vi "cRIO MC Test.vi"() -> ()   [LabVIEW 2009]
uses:
  Remote Control/Motor Command.ctl
  <vilib>/Platform/TimedLoop/XDataNode/wakeup.ctl
  <vilib>/Platform/TimedLoop/XDataNode/XDNodeRunTimeDep.lvlib
  <vilib>/Platform/TimedLoop/XDataNode/nitl_modes.ctl
  <vilib>/Platform/TimedLoop/XDataNode/timing_clust.ctl
  <vilib>/Platform/TimedLoop/XDataNode/XDataNode.xnode
  <vilib>/Platform/TimedLoop/XDataNode/loadlvalarms.vi
  TypeDefs/State Machine/Main State.ctl
  TypeDefs/Queue TypeDefs/Motor State.ctl
  TypeDefs/Queue TypeDefs/Motor Instruction.ctl
  Remote Control/Message Type.ctl
  Remote Control/Control Message.ctl
panel:
  in  "STOP":bool
  out "VI":bool
  in  "MC CMD \n INPUT":T1
  out "UDP HB":bool
  out "Main HB":bool
  out "Motor State":T2=enum."Initialize"
  out "MC HB":bool
  in  "GO":bool
  out "Saftey OFF":bool
  in  "Control Message":T3
  out "Motor Queue":refnum<queue>
  out "RC/!Run":bool
  out "Main State":T4
  in  "RC Command Buffer":T1
  in  "Motors Init Complete":bool
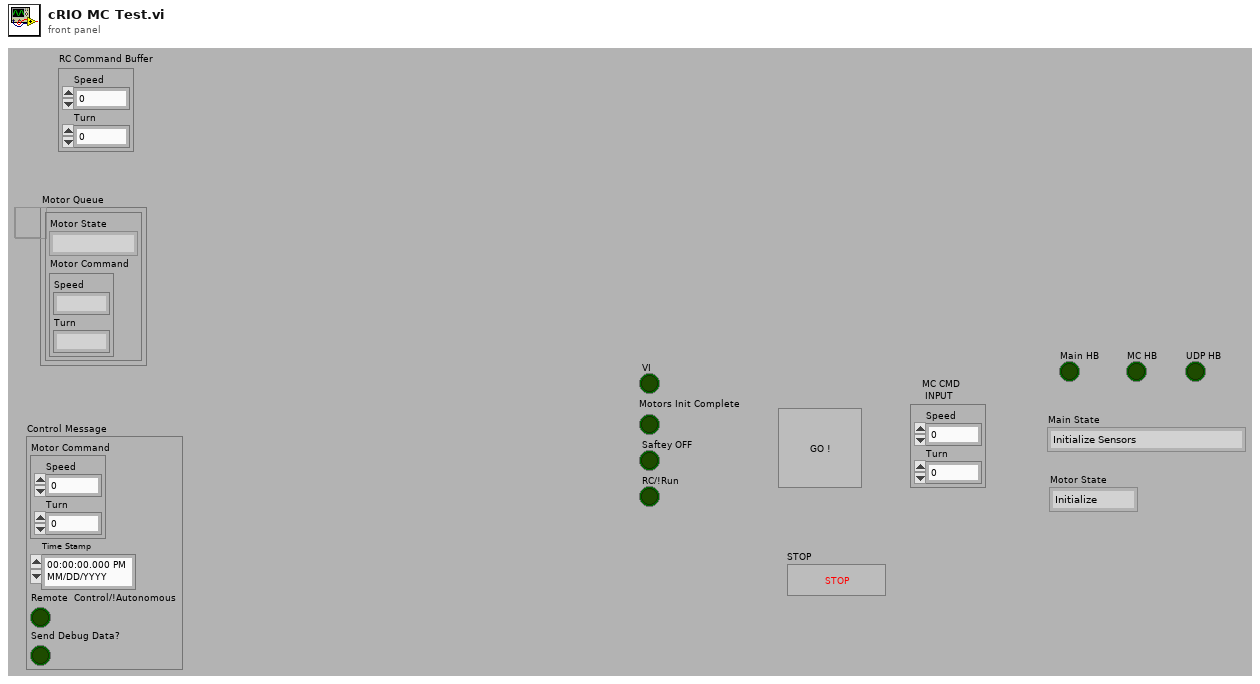
[diagram p1: front panel]
types:
  T1 = typedef "Motor Command.ctl" = cluster{"Speed":i16, "Turn":i16}
  T2 = typedef "Motor State.ctl" = enum16{"Wait", "Initialize", "Check FET", "Run", "Stop"}
  T3 = typedef "Control Message.ctl" = cluster{"Motor Command":T1, "Time Stamp":timestamp, "Remote  Control/!Autonomous":bool, "Send Debug Data?":bool}
  T4 = typedef "Main State.ctl" = enum16{"Initialize Sensors", "Initialize Motors", "Wait for GO", "Run", "Remote Control", "Stop"}
  T5 = typedef "Motor Instruction.ctl" = cluster{"Motor State":T2, "Motor Command":T1}
  T6 = typedef "UDP Base.ctl" = cluster{"UDP Session":refnum<k16>, "UDP Socket Params":T7}
  T7 = typedef "UDP Socket Params.ctl" = cluster{"Local Port":u16, "Read Timeout":i32, "Write Timeout":i32}
  T8 = typedef "XDNodeRunTimeDep.lvlib/timing_clust.ctl" = cluster{"Expected End [f-1]":u64, "Actual End [f-1]":u64, "Finished Late? [f-1]":bool, "Expected End [i-1]":u64, "Actual End [i-1]":u64, "Finished Late? [i-1]":bool, "Expected Start [i]":u64, "Actual Start [i]":u64, "Expected Start [f]":u64, "Actual Start [f]":u64, "Source Name":string, "Structure Name":string, "Period":i64, "Deadline":i64, "Offset":i64, "Start":i64, "Priority":i32, "Timeout":i32, "Mode":T9, "Wakeup Reason":T10, "Error":errorcluster, "Source Type":string, "Secondary Source Type":string, "Global End Time":u64, "Global Start Time":u64, "Frame Duration":u64, "Iteration Duration":u64, "Assigned CPU":i32, "I/O Scan Engine Mode":u32}
  T9 = typedef "XDNodeRunTimeDep.lvlib/nitl_modes.ctl" = enum32{"No Change", "Process missed periods, maintain original phase", "Discard missed periods, maintain original phase", "Process missed periods, ignore original phase", "Discard missed periods, ignore original phase"}
  T10 = typedef "XDNodeRunTimeDep.lvlib/wakeup.ctl" = enum32{"Normal", "Aborted", "Asynchronous wakeup", "Timing source error", "Timed loop error", "Timeout"}
  T11 = typedef "Message Type.ctl" = enum16{"Motor Command", "Debug Data"}
  T12 = typedef "UDP Network Location.ctl" = cluster{"IP Address":string, "Port":u16}
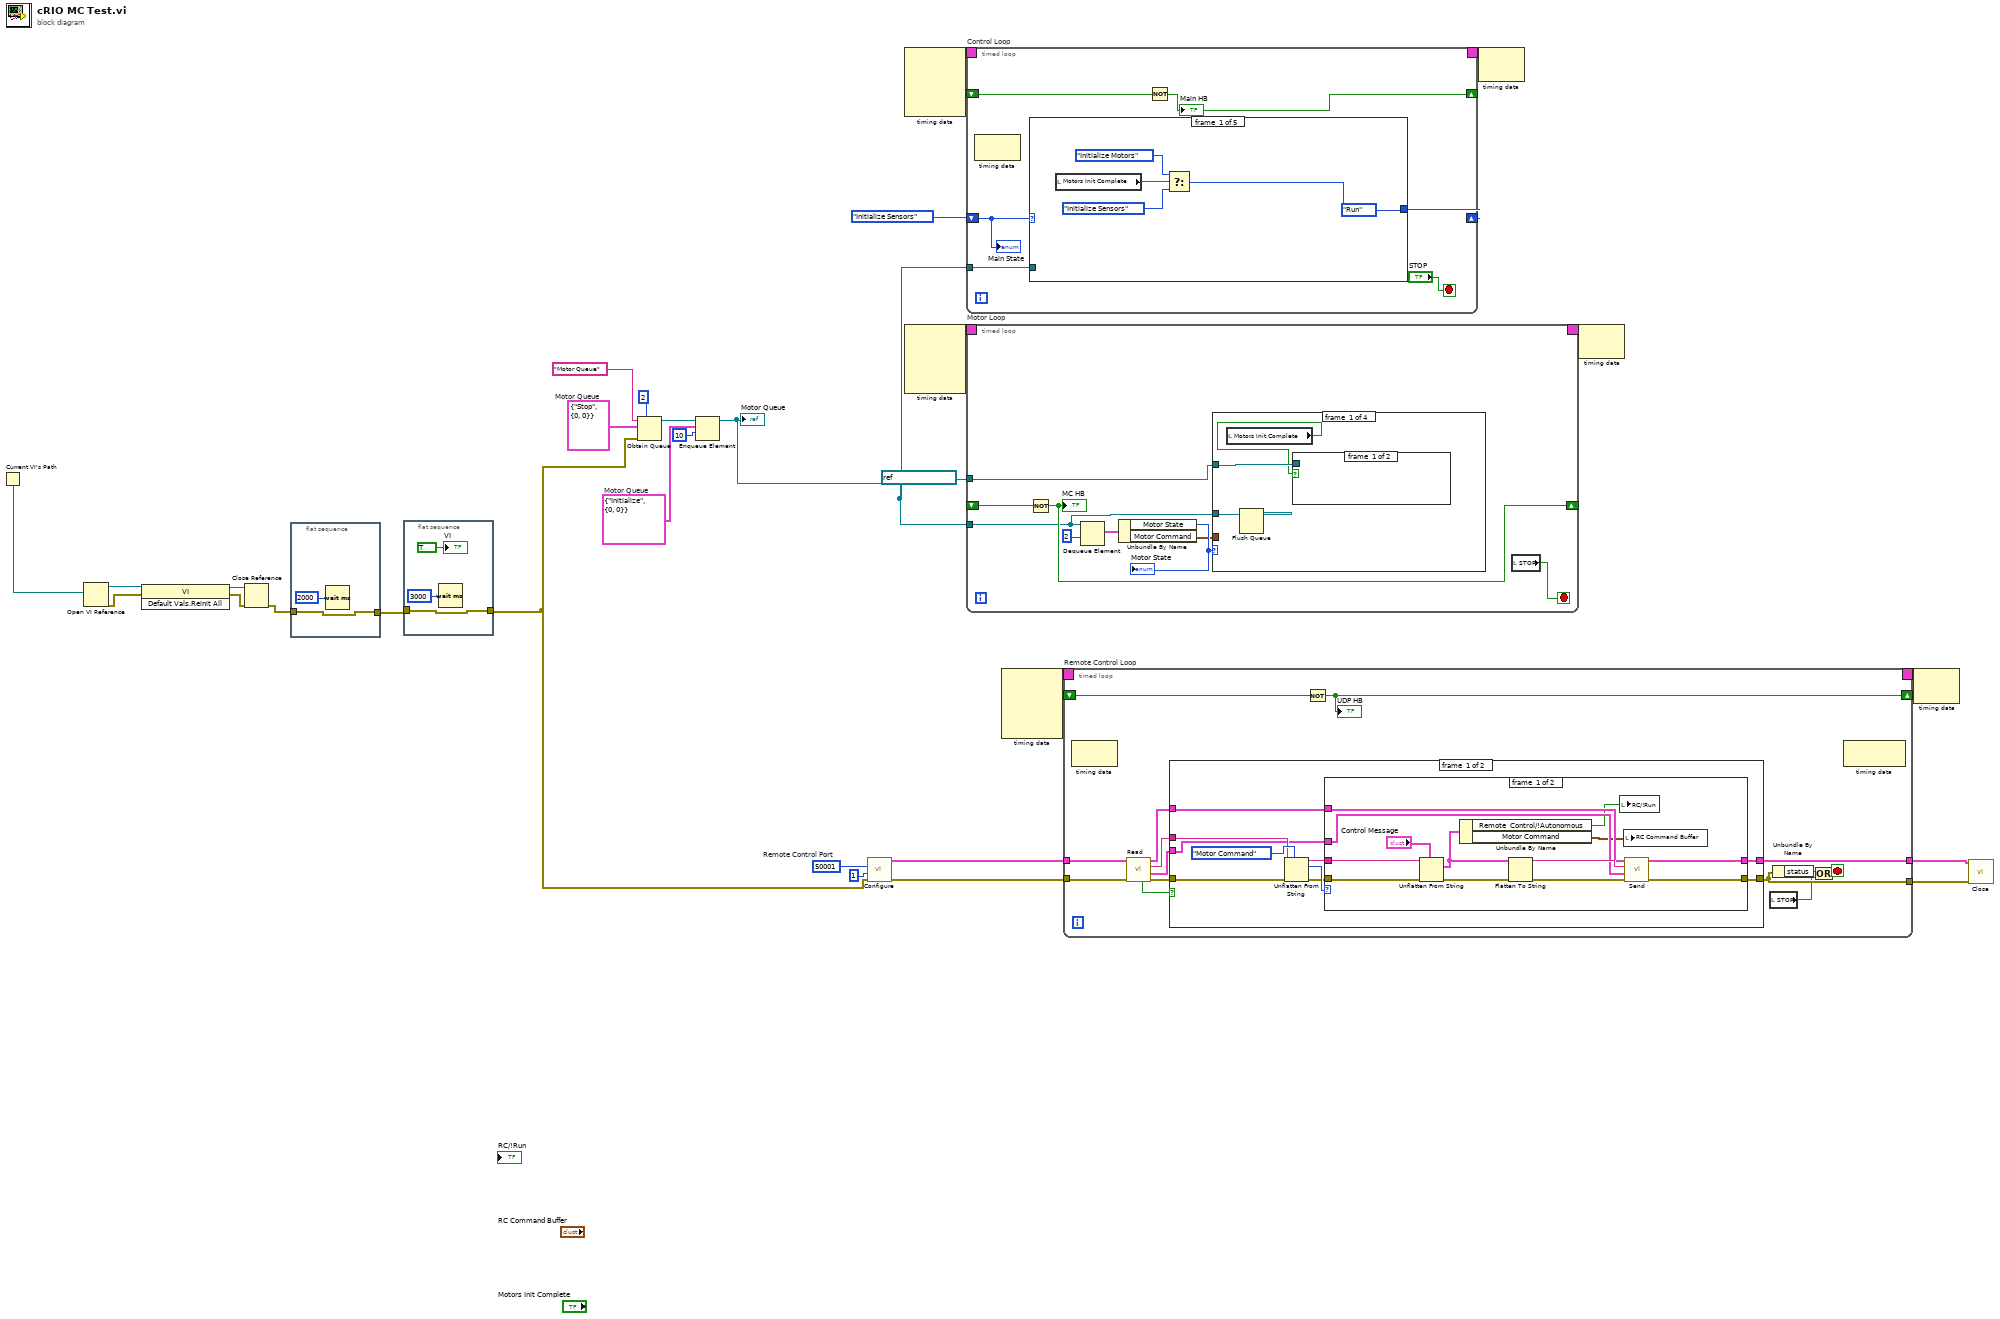
[diagram p0: block diagram]
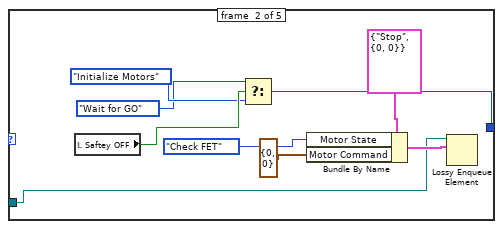
[diagram p4: hidden frame]
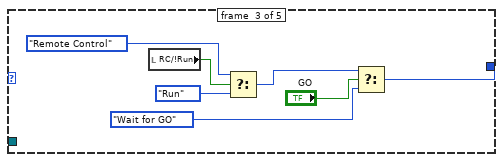
[diagram p5: hidden frame]
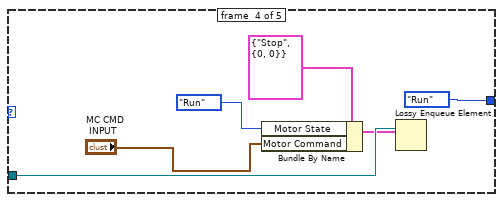
[diagram p6: hidden frame]
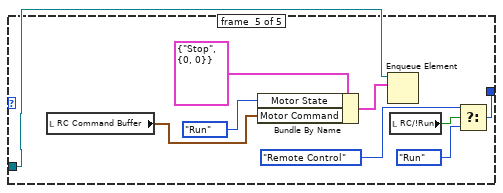
[diagram p7: hidden frame]
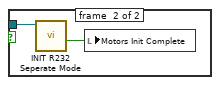
[diagram p8: hidden frame]
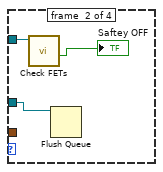
[diagram p9: hidden frame]
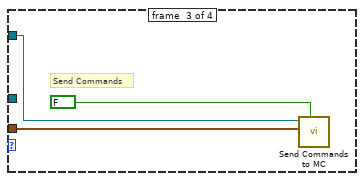
[diagram p10: hidden frame]
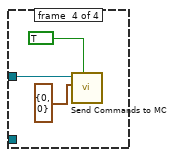
[diagram p11: hidden frame]
diagram:
  w5 = T5 {"Motor State"=enum."Initialize", "Motor Command"={"Speed"=0, "Turn"=0}}  # Motor Queue
  w6 = T5 {"Motor State"=enum."Stop", "Motor Command"={"Speed"=0, "Turn"=0}}  # Motor Queue
  w19 = u16 50001  # Remote Control Port
  n1 = Current VI's Path() -> (path=w14:path)
  n2 = Open VI Reference(vi path=w14) -> (vi reference=w12:refnum<vi>, error out=w13:errorcluster)  [unwired: 5 in]
  n3 = invoke class="VI" method="Default Vals.Reinit All"(reference=w12, error in=w13) -> (reference out=w10:refnum<vi>, error out=w11:errorcluster)  [unwired: 1 in, 1 out]
  n4 = Close Reference(reference=w10, error in (no error)=w11) -> (error out=w2:errorcluster)
  n5 = flat-sequence {
    tunnel: w2 -> [w30]
    tunnel: [w30] -> w1
    frame #0 {
      n6 = Wait (ms)(milliseconds to wait=u32 2000) -> ()  [unwired: 1 out]
    }
  }
  n7 = flat-sequence {
    tunnel: w1 -> [w33]
    tunnel: [w33] -> w4
    frame #0 {
      n8 = Wait (ms)(milliseconds to wait=u32 3000) -> ()  [unwired: 1 out]
      "VI" <- TRUE
    }
  }
  n9 = Obtain Queue(max queue size (-1, unlimited)=2, name (unnamed)="Motor Queue", element data type=w6, error in (no error)=w4) -> (queue out=w9:refnum<queue>)  [unwired: 1 in, 2 out]
  n10 = Enqueue Element(queue=w9, element=w5, timeout in ms (-1)=10) -> (queue out=w17:refnum<queue>)  [unwired: 1 in, 2 out]
  "Motor Queue" <- w17
  n11 = call "Configure.vi"("error in"=w4, "Read Timeout"=1, "Local Port"=w19) -> ("error out"=w22:errorcluster, "UDP Base out"=w23:T6)  [unwired: 7 in]
  n12 = node-c288() -> (w27:T8)  [unwired: 4 in]
  n13 = node-c288() -> (w29:T8)  [unwired: 4 in]
  n14 = timed-loop "Control Loop" {
    timing: w27 -> [_]
    timing-out: [_] -> w26
    tunnel: w17 -> [w40]
    shift-right: [w39] -> _
    shift-left: Main_State."Initialize Sensors" ("Main State") -> [w35]
    shift-right: [w37] -> _
    shift-left: _ -> [w38]
    stop <- "STOP" stop-if-true
    n15 = node-c288() -> ()  [unwired: 1 in, 1 out]
    n16 = case shown="\"Initialize Motors\"" w35 {
      tunnel: w40 -> [_ w47 _ w63 w69]
      tunnel: [w42 w53 w56 Main_State."Run" ("Main State") w68] -> w39
      frame #0 {
        (unwired) Main_State."Run" ("Main State")
        n17 = local read "Motors Init Complete"() -> (w43:bool)
        n18 = Select(t=Main_State."Initialize Motors" ("Main State"), s=w43, f=Main_State."Initialize Sensors" ("Main State")) -> (s? t:f=w42:T4)
      }
      frame #1 {
        n19 = local read "Saftey OFF"() -> (w54:bool)
        n20 = Select(t=Main_State."Wait for GO" ("Main State"), s=w54, f=Main_State."Initialize Motors" ("Main State")) -> (s? t:f=w53:T4)
        n21 = Bundle By Name(cluster=T5 {"Motor State"=enum."Stop", "Motor Command"={"Speed"=0, "Turn"=0}} ("element"), "Motor State"=Motor_State."Check FET", "Motor Command"=T1 {"Speed"=0, "Turn"=0}) -> (w49:T5)
        n22 = Lossy Enqueue Element(queue=w47, element=w49) -> ()  [unwired: 1 in, 4 out]
      }
      frame #2 {
        n23 = local read "RC/!Run"() -> (w58:bool)
        n24 = Select(t=Main_State."Remote Control" ("Main State"), s=w58, f=Main_State."Run" ("Main State")) -> (s? t:f=w57:T4)
        n25 = Select(t=w57, s="GO", f=Main_State."Wait for GO" ("Main State")) -> (s? t:f=w56:T4)
      }
      frame #3 {
        n26 = Bundle By Name(cluster=T5 {"Motor State"=enum."Stop", "Motor Command"={"Speed"=0, "Turn"=0}} ("element"), "Motor State"=Motor_State."Run", "Motor Command"="MC CMD \n INPUT") -> (w62:T5)
        n27 = Lossy Enqueue Element(queue=w63, element=w62) -> ()  [unwired: 1 in, 4 out]
      }
      frame #4 {
        n28 = local read "RC Command Buffer"() -> (w76:T1)
        n29 = Bundle By Name(cluster=T5 {"Motor State"=enum."Stop", "Motor Command"={"Speed"=0, "Turn"=0}} ("element"), "Motor State"=Motor_State."Run", "Motor Command"=w76) -> (w72:T5)
        n30 = Enqueue Element(queue=w69, element=w72) -> ()  [unwired: 2 in, 3 out]
        n31 = local read "RC/!Run"() -> (w75:bool)
        n32 = Select(t=Main_State."Remote Control" ("Main State"), s=w75, f=Main_State."Run" ("Main State")) -> (s? t:f=w68:T4)
      }
    }
    n33 = Not(x=w38) -> (.not. x?=w37:bool)
    "Main HB" <- w37
    "Main State" <- w35
  }
  n34 = timed-loop "Motor Loop" {
    timing: w29 -> [_]
    timing-out: [_] -> w28
    tunnel: w17 -> [w78]
    shift-right: [w82] -> _
    shift-left: _ -> [w81]
    tunnel: refnum<visa-resource-name> "ASRL1::INSTR" ("MC VISA resource") -> [w80]
    stop <- w79 stop-if-true
    n35 = Not(x=w81) -> (.not. x?=w82:bool)
    "MC HB" <- w82
    n36 = Dequeue Element(queue=w78, timeout in ms (-1)=2) -> (element=w86:T5)  [unwired: 1 in, 3 out]
    n37 = Unbundle By Name(w86) -> ("Motor State"=w85:T2, "Motor Command"=w84:T1)
    "Motor State" <- w85
    n38 = case shown="\"Check FET\"" w85 {
      tunnel: w80 -> [w89 w94 w97 w100]
      tunnel: w84 -> [_ _ w95 _]
      tunnel: w78 -> [w88 w93 _ _]
      frame #0 {
        n39 = local read "Motors Init Complete"() -> (w87:bool)
        n40 = Flush Queue(queue=w88) -> ()  [unwired: 1 in, 3 out]
        n41 = case shown="False" w87 {
          tunnel: w89 -> [_ w91]
          frame #0 {
          }
          frame #1 {
            n42 = call "INIT R232 Seperate Mode.vi"("MC VISA resource in"=w91) -> ("MC Init Complete"=w90:bool)  [unwired: 8 in, 2 out]
            n43 = local write "Motors Init Complete"(w90) -> ()
          }
        }
      }
      frame #1 {
        n44 = call "Check FETs.vi"("MC VISA resource in"=w94) -> ("FETs on?"=→"Saftey OFF":bool)  [unwired: 6 in, 4 out]
        n45 = Flush Queue(queue=w93) -> ()  [unwired: 1 in, 3 out]
      }
      frame #2 {
        # "Send Commands"
        n46 = call "Send Commands to MC.vi"("Pause Motors"=FALSE, "Motor Command"=w95, "MC refrence in"=w97) -> ()  [unwired: 4 in, 2 out]
      }
      frame #3 {
        n47 = call "Send Commands to MC.vi"("Pause Motors"=TRUE, "Motor Command"=T1 {"Speed"=0, "Turn"=0}, "MC refrence in"=w100) -> ()  [unwired: 4 in, 2 out]
      }
    }
    n48 = local read "STOP"() -> (w79:bool)
  }
  n49 = node-c288() -> (w25:T8)  [unwired: 4 in]
  n50 = timed-loop "Remote Control Loop" {
    tunnel: w23 -> [w114]
    tunnel: w22 -> [w113]
    tunnel: [w116] -> w20
    tunnel: [w115] -> w21
    timing: w25 -> [_]
    timing-out: [_] -> w24
    shift-right: [w105] -> _
    shift-left: _ -> [w106]
    stop <- w104 stop-if-true
    n51 = node-c288() -> ()  [unwired: 1 in, 1 out]
    n52 = call "Read.vi"("error in (no error)"=w113, "UDP Base in"=w114) -> ("error out"=w111:errorcluster, "Network Location"=w108:T12, "Receive Data"=w110:string, "UDP Base out"=w112:T6, "Timeout"=w109:bool)  [unwired: 4 in, 1 out]
    n53 = case shown="False" w109 {
      tunnel: [w126 w144] -> w116
      tunnel: [w125 w145] -> w115
      tunnel: w112 -> [w122 w145]
      tunnel: w111 -> [w121 w144]
      tunnel: w110 -> [w120 _]
      tunnel: w108 -> [w119 _]
      frame #0 {
        n54 = Unflatten From String(type=Message_Type."Motor Command" ("Message Type"), binary string=w120, error in (no error)=w121) -> (rest of the binary string=w123:string, value=w127:T11, error out=w124:errorcluster)  [unwired: 2 in]
        n55 = case shown="\"Motor Command\", Default" w127 {
          tunnel: [w135 w143] -> w126
          tunnel: [w136 w142] -> w125
          tunnel: w124 -> [w141 w143]
          tunnel: w123 -> [w140 _]
          tunnel: w122 -> [w133 w142]
          tunnel: w119 -> [w131 _]
          frame #0 {
            n56 = Unflatten From String(type="Control Message", binary string=w140, error in (no error)=w141) -> (value=w132:T3, error out=w139:errorcluster)  [unwired: 2 in, 1 out]
            n57 = Unbundle By Name(w132) -> ("Remote  Control/!Autonomous"=w129:bool, "Motor Command"=w130:T1)
            n58 = Flatten To String(anything=w132, error in (no error)=w139) -> (data string=w134:string, error out=w137:errorcluster)  [unwired: 2 in, 1 out]
            n59 = local write "RC/!Run"(w129) -> ()
            n60 = local write "RC Command Buffer"(w130) -> ()
            n61 = call "Send.vi"("error in (no error)"=w137, "Destination Location"=w131, "Send Data"=w134, "UDP Base in"=w133) -> ("error out"=w135:errorcluster, "UDP Base out"=w136:T6)  [unwired: 5 in, 1 out]
          }
          frame #1 {
          }
        }
      }
      frame #1 {
      }
    }
    n62 = Not(x=w106) -> (.not. x?=w105:bool)
    "UDP HB" <- w105
    n63 = local read "STOP"() -> (w103:bool)
    n64 = Unbundle By Name(w116) -> ("status"=w107:bool)
    n65 = Or(x=w107, y=w103) -> (x .or. y?=w104:bool)
    n66 = node-c288() -> ()  [unwired: 1 in, 1 out]
  }
  n67 = node-c288(w26) -> ()  [unwired: 1 out]
  n68 = node-c288(w28) -> ()  [unwired: 1 out]
  n69 = node-c288(w24) -> ()  [unwired: 1 out]
  n70 = call "Close.vi"("error in (no error)"=w20, "Cluster of class private data"=w21) -> ()  [unwired: 9 in, 1 out]
